vi "JoystickRefNums.vi"() -> (0 "Joysticks":T1={"Driver Controller"={"Device"=enum."USB 1"}, "Operator Controller"={"Device"=enum."USB 1"}})   [LabVIEW 2017]
uses:
  TypeDefs/RobotComponents/RobotJoysticks.ctl
  <vilib>/Rock Robotics/WPI/Joystick/WPI_JoystickDevRef.ctl
  <vilib>/Rock Robotics/WPI/Joystick/WPI_JoystickDeviceEnum.ctl
  <vilib>/Rock Robotics/WPI/Utilities/WPI_GetSetVariantRefNum.vi
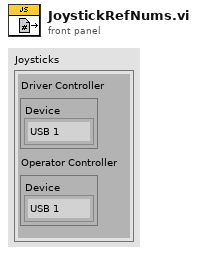
[diagram p1: front panel]
types:
  T1 = typedef "RobotJoysticks.ctl" = cluster{"Driver Controller":T2, "Operator Controller":T2}
  T2 = typedef "WPI_JoystickDevRef.ctl" = cluster{"Device":T3}
  T3 = typedef "WPI_JoystickDeviceEnum.ctl" = enum16{"USB 0", "USB 1", "USB 2", "USB 3", "USB 4", "USB 5"}
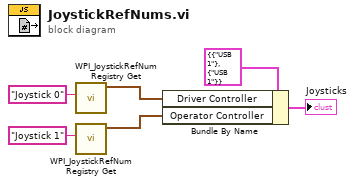
[diagram p0: block diagram]
diagram:
  n1 = call <vilib>:"WPI_JoystickRefNum Registry Get.vi"("refnum name"="Joystick 0") -> ("JoystickDevRef"=w2:T2)  [unwired: 9 in, 1 out]
  n2 = call <vilib>:"WPI_JoystickRefNum Registry Get.vi"("refnum name"="Joystick 1") -> ("JoystickDevRef"=w1:T2)  [unwired: 9 in, 1 out]
  n3 = Bundle By Name(cluster=T1 {"Driver Controller"={"Device"=enum."USB 1"}, "Operator Controller"={"Device"=enum."USB 1"}} ("Joysticks"), "Driver Controller"=w2, "Operator Controller"=w1) -> (→"Joysticks":T1)
